vi "ChangeValuePopup.vi"(0 "Enable":bool=TRUE, 1 "Device description":string, 2 "Initial value":dbl, 5 "error in (no error)":errorcluster) -> (17 "Device value":dbl format="%#g", 18 "OK":bool, 19 "error out":errorcluster)   [LabVIEW 2020]
doc: "Displays a standard dialog box that prompts users to enter information, such as a user name and password.\n--------------------\n\nThis Express VI is configured as follows:\n\nMessage to Display to the User:Please select a new value\nThe inputs are: \nNumber: Device value"
panel:
  in  "Device value":dbl format="%#.6g"
  out "String":string="Please select a new value"
  in  "Cancel":bool
  in  "OK2":bool
  in  "OK1":bool
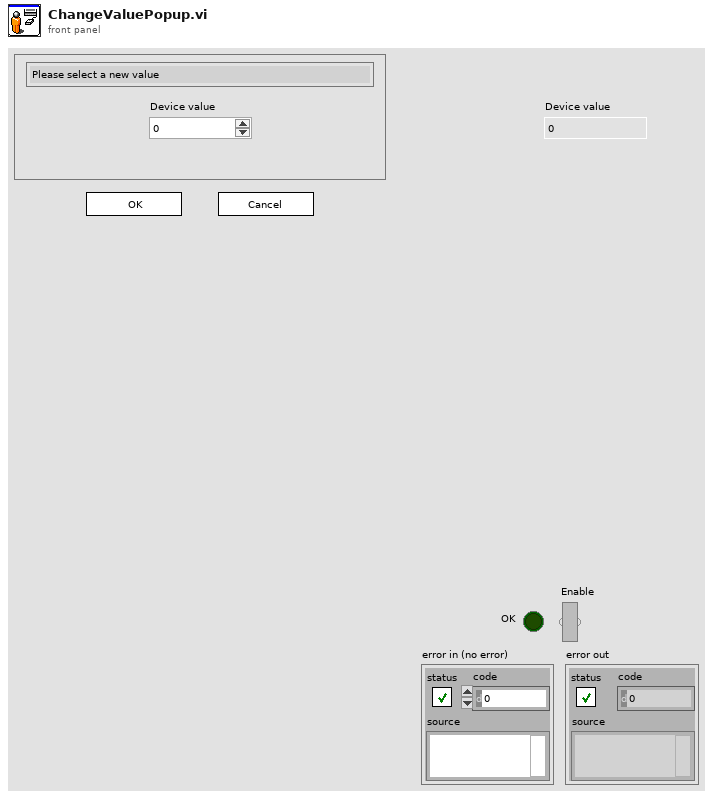
[diagram p1: front panel]
types:
  T1 = cluster{"Input Name":string, "Input Data Type":i32}[]
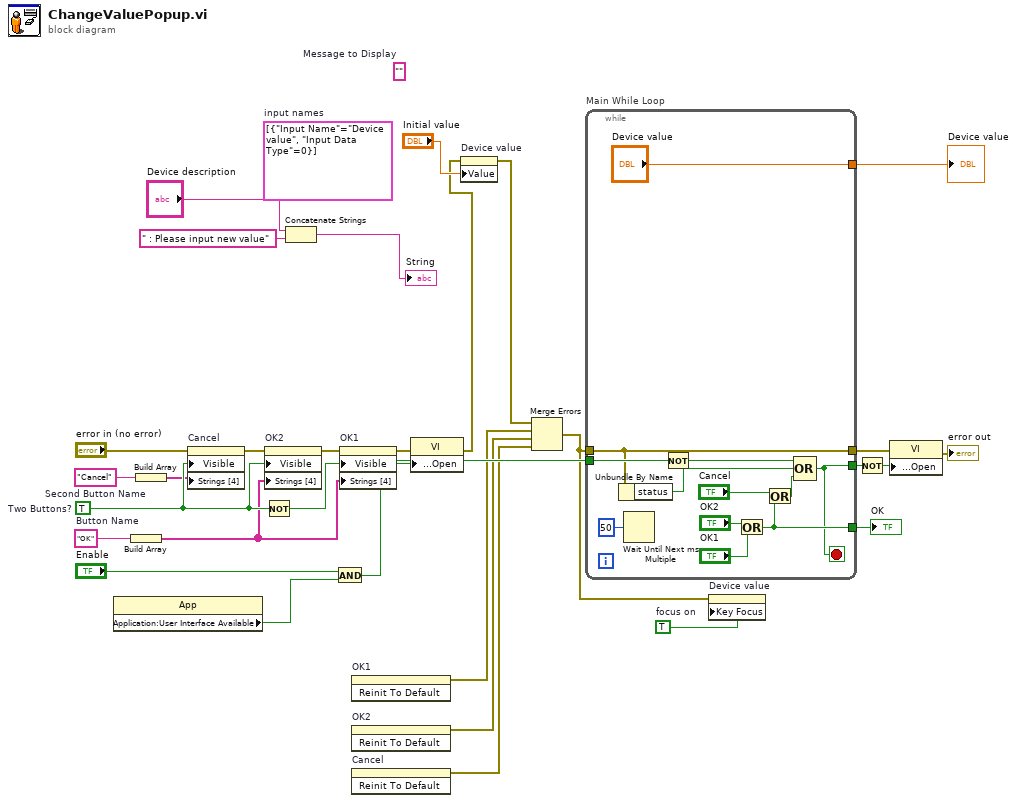
[diagram p0: block diagram]
diagram:
  w11 = TRUE  # focus on
  (unwired) T1 [{"Input Name"="Device value", "Input Data Type"=0}]  # input names
  w22 = "Cancel"  # Second Button Name
  w20 = "OK"  # Button Name
  (unwired) ""  # Message to Display
  w30 = TRUE  # Two Buttons?
  n1 = property class="App"() -> ("Application:User Interface Available"=w13:bool)  [unwired: 2 in, 2 out]
  n2 = Build Array(w20) -> (w21:string[])
  n3 = Build Array(w22) -> (w23:string[])
  n4 = property on="Cancel" class="Bool"(error in="error in (no error)", "Visible"=w30, "Strings [4]"=w23) -> (error out=w27:errorcluster)  [unwired: 1 in, 1 out]
  n5 = Not(x=w30) -> (.not. x?=w28:bool)
  n6 = property on="OK2" class="Bool"(error in=w27, "Visible"=w30, "Strings [4]"=w21) -> (error out=w26:errorcluster)  [unwired: 1 in, 1 out]
  n7 = Concatenate Strings("Device description", " : Please input new value" ("string")) -> (→"String":string)
  n8 = And(x="Enable", y=w13) -> (x .and. y?=w14:bool)
  n9 = property on="OK1" class="Bool"(error in=w26, "Visible"=w28, "Strings [4]"=w21) -> (error out=w19:errorcluster)  [unwired: 1 in, 1 out]
  n10 = invoke on="OK1" class="Bool" method="Reinit To Default"() -> (error out=w3:errorcluster)  [unwired: 3 in, 2 out]
  n11 = invoke on="OK2" class="Bool" method="Reinit To Default"() -> (error out=w2:errorcluster)  [unwired: 3 in, 2 out]
  n12 = invoke on="Cancel" class="Bool" method="Reinit To Default"() -> (error out=w1:errorcluster)  [unwired: 3 in, 2 out]
  n13 = property class="VI"(error in=w19, "Front Panel Window:Open"=w14) -> (error out=w7:errorcluster)  [unwired: 1 in, 1 out]
  n14 = property on="Device value" class="DigNum (strict)"(error in=w7, "Value"="Initial value") -> (error out=w6:errorcluster)  [unwired: 1 in, 1 out]
  n15 = Merge Errors(w6, w3, w2, w1) -> (w4:errorcluster)
  n16 = while "Main While Loop" {
    tunnel: [w39] -> w29
    tunnel: w14 -> [w37]
    tunnel: [w35] -> w24
    tunnel: w4 -> [w34]
    tunnel: [w34] -> w17
    tunnel: ["Device value"] -> w12
    stop <- w35 stop-if-true
    n17 = Unbundle By Name(w34) -> ("status"=w32:bool)
    n18 = Wait Until Next ms Multiple(millisecond multiple=u32 50) -> ()  [unwired: 1 out]
    n19 = Not(x=w37) -> (.not. x?=w36:bool)
    n20 = Or(x="OK2", y="OK1") -> (x .or. y?=w39:bool)
    n21 = Or(x="Cancel", y=w39) -> (x .or. y?=w33:bool)
    n22 = Compound Arithmetic op=OR(w36, w32, w33) -> (w35:bool)
  }
  "OK" <- w29
  "Device value" <- w12
  n23 = property on="Device value" class="DigNum (strict)"(error in=w4, "Key Focus"=w11) -> ()  [unwired: 1 in, 2 out]
  n24 = Not(x=w24) -> (.not. x?=w25:bool)
  n25 = property class="VI"(error in=w17, "Front Panel Window:Open"=w25) -> (error out=→"error out":errorcluster)  [unwired: 1 in, 1 out]
